vi "AO.vi"() -> ()   [LabVIEW 2021]
uses:
  <vilib>/rvi/Emulation/niFpgaGetClockAttributes.vi
  <vilib>/rvi/Emulation/niFpgaSctlEmulationGetInTimedLoop.vi
  <vilib>/rvi/Emulation/niFpgaEmulationReportErrorSimple.vi
  <vilib>/rvi/Emulation/niFpgaProcessEmulError.vi
  <vilib>/rvi/interface/RandomDataEmulation/niFpgaRandomDataHandleErrors.vi
  <vilib>/rvi/Emulation/niFpgaCriticalErrorInLSC.vi
  <vilib>/rvi/eio/common/nirviEmuTemplateMethod_errors.vi
  <vilib>/rvi/DataTransferAndStorage/Container/XNode/niFpgaContainer.xnode
  <vilib>/rvi/interface/RandomDataEmulation/nirviRandomDataFpgaReadWriteTemplate.vi
  <vilib>/eio/EIONode/EIONode.xnode
panel:
  out "AO: Actual Loop Rate(ticks)":u32
  in  "AO 0":i16
  in  "AO 1":i16
  in  "AO 2":i16
  in  "AO 3":i16
  in  "AO 4":i16
  in  "AO 5":i16
  in  "AO 6":i16
  in  "AO 7":i16
  in  "AO Loop Timer(Ticks)":u32
  out "AO Buffer Underflow?":bool
  in  "AO Buffer Enable":u8 format="%08b"
  in  "AO Enable":bool
  # "Analog Output"
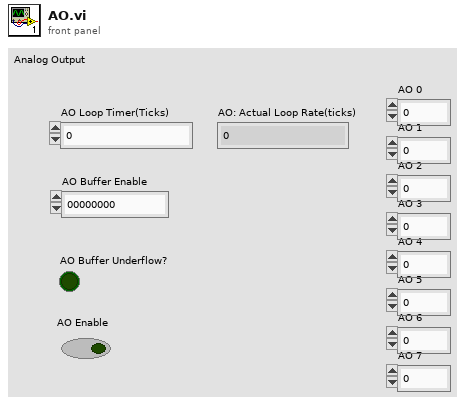
[diagram p1: front panel]
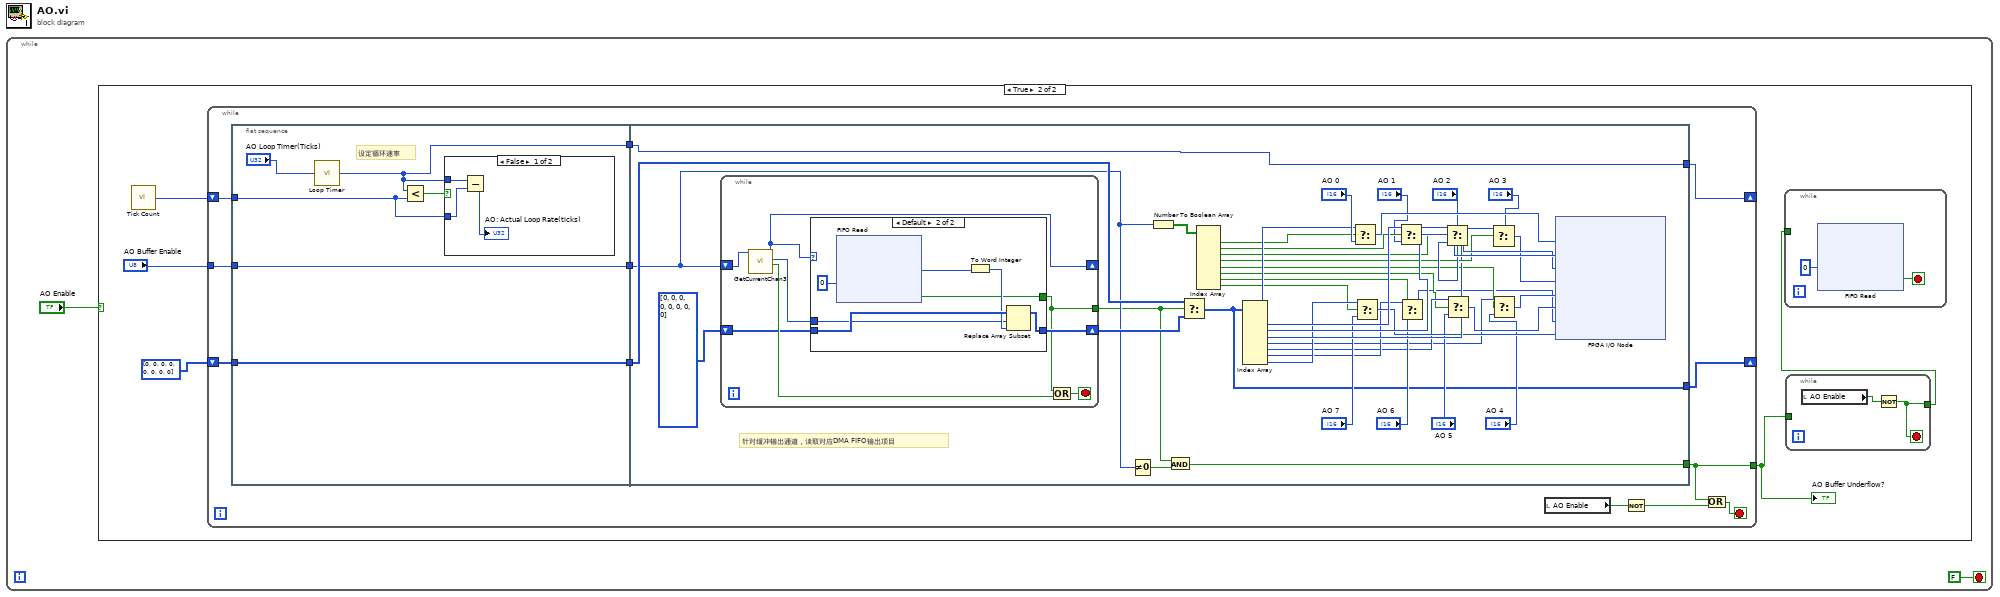
[diagram p0: block diagram]
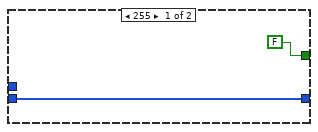
[diagram p4: hidden frame]
diagram:
  n1 = while {
    stop <- FALSE stop-if-true
    n2 = case shown="True" "AO Enable" {
      frame False {
      }
      frame True {
        n3 = call "Tick Count"() -> ("Tick Count(Ticks)"=w7:u32)
        n4 = while {
          shift-right: [w12] -> _
          shift-left: w7 -> [w19]
          tunnel: "AO Buffer Enable" -> [w17]
          shift-right: [w13] -> _
          shift-left: i16[] [0, 0, 0, 0, 0, 0, 0, 0] -> [w14]
          tunnel: [w8] -> w4
          stop <- w10 stop-if-true
          n5 = flat-sequence {
            tunnel: w19 -> [w23]
            tunnel: [w22] -> w18
            tunnel: w17 -> [w22]
            tunnel: [w21] -> w16
            tunnel: [w20] -> w15
            tunnel: w14 -> [w20]
            tunnel: w18 -> [w65]
            tunnel: w16 -> [w31]
            tunnel: w15 -> [w68]
            tunnel: [w32] -> w13
            tunnel: [w31] -> w12
            tunnel: [w30] -> w8
            frame #0 {
              # "设定循环速率"
              n6 = call "Loop Timer"("Count(Ticks)"="AO Loop Timer(Ticks)") -> ("Tick Count(Ticks)"=w21:u32)
              n7 = Less?(x=w21, y=w23) -> (x < y?=w25:bool)
              n8 = case shown="False" w25 {
                tunnel: w21 -> [w28 _]
                tunnel: w23 -> [w27 _]
                frame False {
                  n9 = Subtract(x=w28, y=w27) -> (x-y=→"AO: Actual Loop Rate(ticks)":u32)
                }
                frame True {
                  # "overflow"
                }
              }
            }
            frame #1 {
              # "针对缓冲输出通道，读取对应DMA FIFO输出项目"
              n10 = while {
                shift-right: [w72] -> w69
                shift-left: i16[] [0, 0, 0, 0, 0, 0, 0, 0] -> [w76]
                shift-right: [w73] -> _
                shift-left: w65 -> [w74]
                tunnel: [w71] -> w64
                stop <- w77 stop-if-true
                n11 = call "GetCurrentChan3.vi"("AI Select In"=w74) -> ("Stop Loop"=w78:bool, "Current Channel"=w75:u8, "AI Select Out"=w73:u8)  [unwired: 8 in]
                n12 = case shown="Default" w73 {
                  tunnel: w76 -> [w79 w85]
                  tunnel: [w79 w84] -> w72
                  tunnel: [FALSE ("Empty") w81] -> w71
                  tunnel: w75 -> [_ w82]
                  frame 255 {
                  }
                  frame Default {
                    n13 = xnode ("FIFO Read")("Timeout"=0) -> ("Element"=w86:u32, "Timed Out?"=w81:bool)  [unwired: 1 in, 1 out]
                    n14 = To Word Integer(number=w86) -> (16bit integer=w83:i16)
                    n15 = Replace Array Subset(array=w85, new element=w83, index=w82) -> (w84:i16[])
                  }
                }
                n16 = Or(x=w71, y=w78) -> (x .or. y?=w77:bool)
              }
              n17 = Not Equal To 0?(x=w65) -> (x != 0?=w66:bool)
              n18 = Number To Boolean Array(number=w65) -> (Boolean array=w67:bool[])
              n19 = And(x=w64, y=w66) -> (x .and. y?=w30:bool)
              n20 = Select(t=w68, s=w64, f=w69) -> (s? t:f=w32:i16[])
              n21 = Index Array(array=w67) -> (element #1=w57:bool, element #2=w56:bool, element #3=w55:bool, element #4=w51:bool, element #5=w33:bool, element #6=w34:bool, element #7=w35:bool, element #8=w46:bool)  [unwired: 8 in]
              n22 = Index Array(array=w32) -> (element #1=w62:i16, element #2=w61:i16, element #3=w58:i16, element #4=w49:i16, element #5=w36:i16, element #6=w37:i16, element #7=w38:i16, element #8=w47:i16)  [unwired: 8 in]
              n23 = Select(t=w62, s=w57, f="AO 0") -> (s? t:f=w60:i16)
              n24 = Select(t=w47, s=w46, f="AO 7") -> (s? t:f=w44:i16)
              n25 = Select(t=w61, s=w56, f="AO 1") -> (s? t:f=w59:i16)
              n26 = Select(t=w38, s=w35, f="AO 6") -> (s? t:f=w29:i16)
              n27 = Select(t=w58, s=w55, f="AO 2") -> (s? t:f=w52:i16)
              n28 = Select(t=w37, s=w34, f="AO 5") -> (s? t:f=w41:i16)
              n29 = Select(t=w49, s=w51, f="AO 3") -> (s? t:f=w48:i16)
              n30 = Select(t=w36, s=w33, f="AO 4") -> (s? t:f=w39:i16)
              n31 = xnode "FPGA I/O Node"("Connector0/AO0"=w60, "Connector0/AO1"=w59, "Connector0/AO2"=w52, "Connector0/AO3"=w48, "Connector0/AO4"=w39, "Connector0/AO5"=w41, "Connector0/AO6"=w29, "Connector0/AO7"=w44) -> ()  [unwired: 8 in, 8 out]
            }
          }
          n32 = local read "AO Enable"() -> (w9:bool)
          n33 = Not(x=w9) -> (.not. x?=w11:bool)
          n34 = Or(x=w8, y=w11) -> (x .or. y?=w10:bool)
        }
        "AO Buffer Underflow?" <- w4
        n35 = while {
          tunnel: w4 -> [_]
          tunnel: [w90] -> w3
          stop <- w90 stop-if-true
          n36 = local read "AO Enable"() -> (w91:bool)
          n37 = Not(x=w91) -> (.not. x?=w90:bool)
        }
        n38 = while {
          tunnel: w3 -> [_]
          stop <- w88 stop-if-true
          n39 = xnode ("FIFO Read")("Timeout"=0) -> ("Timed Out?"=w88:bool)  [unwired: 1 in, 2 out]
        }
      }
    }
  }
